vi "DynamixelCountingPlane.vi"(9 "Motors Read Correctly":bool[](array[boolean]), 10 "Dynamixel Cycles":T1, 11 "Dynamixel Read Positions":dbl[](array[numeric])) -> (2 "Updated Dynamixle Cycles":T1)   [LabVIEW 2013]
doc: "This VI takes the Dynamixel positions, compares them against the old positions, and tests whether that difference merits a change in cycle. If the position jumps high up or high down that indicates the motor crossed the line from 360-0 or 0-360, depending on the sign of the change. This updates the cycle count variable. It also changes the 'motor read correctly' value for the motors."
uses:
  Data/TypeDefs/DynamixelCycleTracker.ctl
panel:
  out "Change for Main":i32
  out "Change for Jib":i32
  out "Change for Rudder":i32
  out "New Main position":dbl
  out "Old Main position":dbl
  out "New Jib position":dbl
  out "Old Jib position":dbl
  out "New Rudder position":dbl
  out "Old Rudder position":dbl
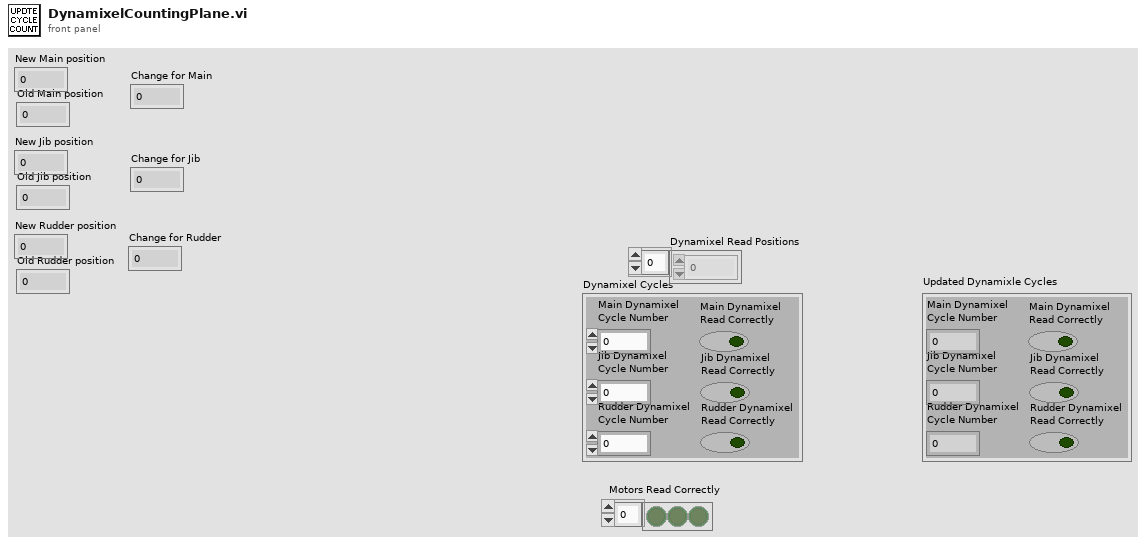
[diagram p1: front panel]
types:
  T1 = typedef "DynamixelCycleTracker.ctl" = cluster{"Main Dynamixel\nCycle Number":i32, "Jib Dynamixel\nCycle Number":i32, "Rudder Dynamixel\nCycle Number":i32, "Main Dynamixel\nRead Correctly":bool, "Jib Dynamixel\nRead Correctly":bool, "Rudder Dynamixel\nRead Correctly":bool}
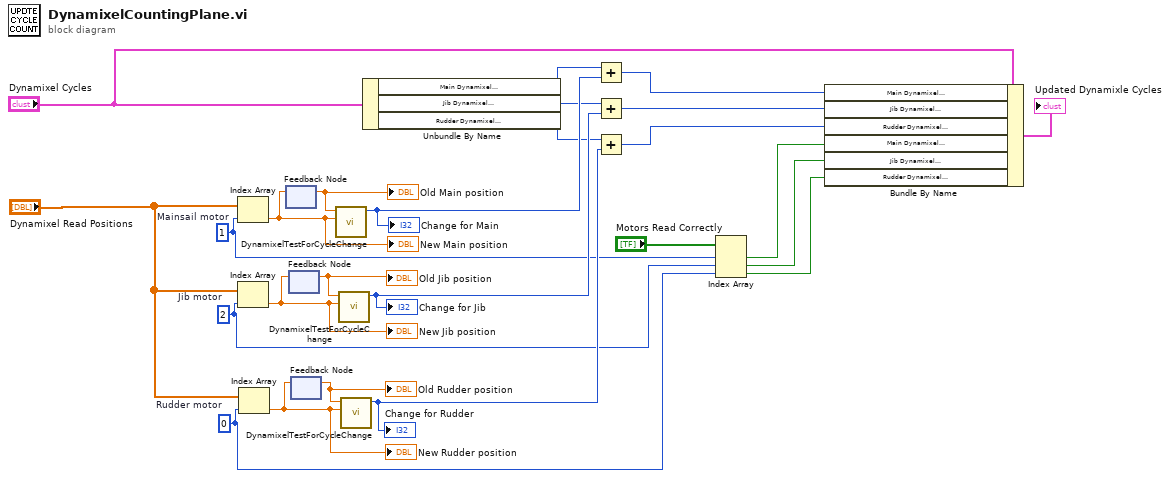
[diagram p0: block diagram]
diagram:
  w6 = 1  # Mainsail motor
  w5 = 2  # Jib motor
  w4 = 0  # Rudder motor
  n1 = Index Array(array="Dynamixel Read Positions", index=w6) -> (element=w12:dbl)
  "New Main position" <- w12
  n2 = Index Array(array="Dynamixel Read Positions", index=w5) -> (element=w9:dbl)
  "New Jib position" <- w9
  n3 = Index Array(array="Dynamixel Read Positions", index=w4) -> (element=w7:dbl)
  "New Rudder position" <- w7
  n4 = feedback #1() -> (w11:dbl)  [unwired: 1 in]
  "Old Main position" <- w11
  n5 = feedback-in #1(w12) -> ()
  n6 = feedback #2() -> (w10:dbl)  [unwired: 1 in]
  "Old Jib position" <- w10
  n7 = feedback-in #2(w9) -> ()
  n8 = feedback #3() -> (w8:dbl)  [unwired: 1 in]
  "Old Rudder position" <- w8
  n9 = feedback-in #3(w7) -> ()
  n10 = call "DynamixelTestForCycleChange.vi"("New position (deg)"=w12, "Old position (deg)"=w11) -> ("Dynamixel Cycle Number"=w24:i32)  [unwired: 9 in]
  "Change for Main" <- w24
  n11 = call "DynamixelTestForCycleChange.vi"("New position (deg)"=w9, "Old position (deg)"=w10) -> ("Dynamixel Cycle Number"=w23:i32)  [unwired: 9 in]
  "Change for Jib" <- w23
  n12 = call "DynamixelTestForCycleChange.vi"("New position (deg)"=w7, "Old position (deg)"=w8) -> ("Dynamixel Cycle Number"=w22:i32)  [unwired: 9 in]
  "Change for Rudder" <- w22
  n13 = Unbundle By Name("Dynamixel Cycles") -> ("Main Dynamixel\nCycle Number"=w19:i32, "Jib Dynamixel\nCycle Number"=w20:i32, "Rudder Dynamixel\nCycle Number"=w21:i32)
  n14 = Add(x=w19, y=w24) -> (x+y=w18:i32)
  n15 = Add(x=w20, y=w23) -> (x+y=w17:i32)
  n16 = Add(x=w21, y=w22) -> (x+y=w16:i32)
  n17 = Index Array(array="Motors Read Correctly", index #1=w6, index #2=w5, index #3=w4) -> (element #1=w3:bool, element #2=w2:bool, element #3=w1:bool)
  n18 = Bundle By Name(cluster="Dynamixel Cycles", "Main Dynamixel\nCycle Number"=w18, "Jib Dynamixel\nCycle Number"=w17, "Rudder Dynamixel\nCycle Number"=w16, "Main Dynamixel\nRead Correctly"=w3, "Jib Dynamixel\nRead Correctly"=w2, "Rudder Dynamixel\nRead Correctly"=w1) -> (→"Updated Dynamixle Cycles":T1)
